vi "Communication Manager.vi"(7 "Load?":bool, 8 "error in":errorcluster, 9 ">>ErrorQ":refnum<queue>, 10 ">>ControllerQ":refnum<queue>, 11 ">>EventHandlers":refnum<user-event>) -> (0 "error out":errorcluster, 3 "Messaging Structures":T1)   [LabVIEW 2020, in "ErrorHandler.lvlib"]
doc: "Stores references to external communication structures for the module"
uses:
  ErrorHandler.lvlib
  Controls/Module Messaging Structures.ctl
  Support/Controls/Project Event Msg.ctl
  Support/Controls/Project Events.ctl
  Controls/Error QMsg.ctl
  Support/Controls/Project Modules.ctl
  Controller/Controls/Controller QMsg.ctl
  Support/Support.lvlib
  Controller/Controller.lvlib
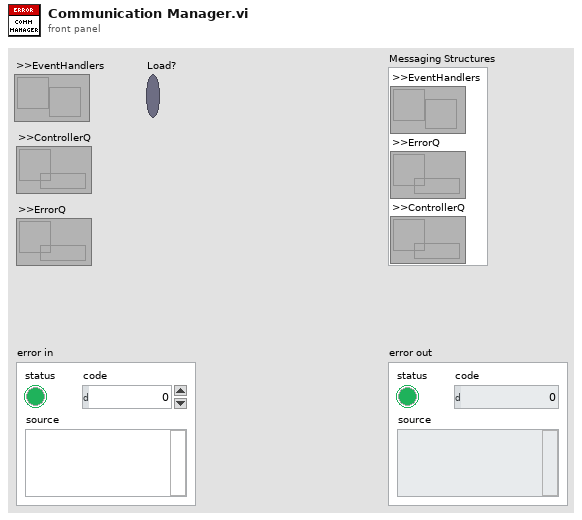
[diagram p1: front panel]
types:
  T1 = typedef "ErrorHandler.lvlib/Module Messaging Structures.ctl" = cluster{">>EventHandlers":refnum<user-event>, ">>ErrorQ":refnum<queue>, ">>ControllerQ":refnum<queue>}
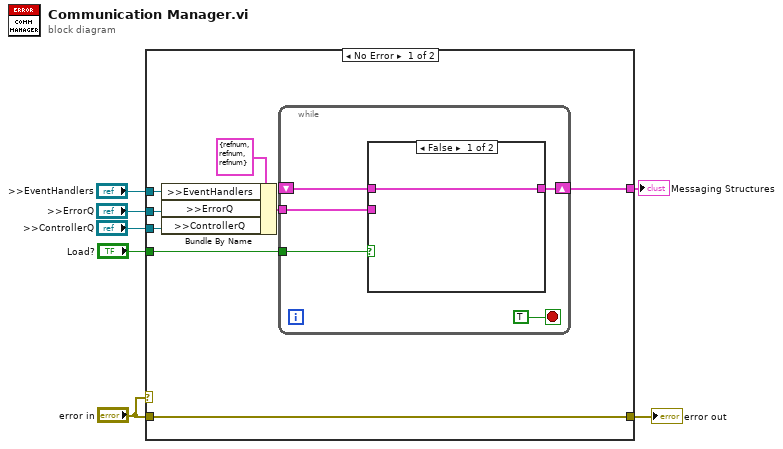
[diagram p0: block diagram]
diagram:
  n1 = case shown="No Error" "error in" {
    tunnel: "error in" -> [w14 w23]
    tunnel: [w14 w23] -> w6
    tunnel: [w10 _] -> w5
    tunnel: ">>ControllerQ" -> [w13 _]
    tunnel: ">>ErrorQ" -> [w12 _]
    tunnel: ">>EventHandlers" -> [w11 _]
    tunnel: "Load?" -> [w8 _]
    frame No Error {
      n2 = Bundle By Name(cluster=T1 {">>EventHandlers"=refnum, ">>ErrorQ"=refnum, ">>ControllerQ"=refnum} ("Messaging Structures"), ">>EventHandlers"=w11, ">>ErrorQ"=w12, ">>ControllerQ"=w13) -> (w9:T1)
      n3 = while {
        shift-right: [w19] -> w10
        shift-left: _ -> [w18]
        tunnel: w9 -> [w17]
        tunnel: w8 -> [w16]
        stop <- TRUE stop-if-true
        n4 = case shown="False" w16 {
          tunnel: [w21 w22] -> w19
          tunnel: w18 -> [w21 _]
          tunnel: w17 -> [_ w22]
          frame False {
          }
          frame True {
          }
        }
      }
    }
    frame Error {
    }
  }
  "error out" <- w6
  "Messaging Structures" <- w5
